vi "Fetch Measurement (Harmonic Distortion).vi"(8 "error in (no error)":errorcluster, 9 "Timeout (20000 ms)":i32=20000, 11 "VISA resource name":refnum<visa-resource-name>) -> (0 "error out":errorcluster, 1 "Frequency Values":dbl[](array[numeric]) format="%#.6g", 2 "Amplitude Values":dbl[](array[numeric]) format="%#.6g", 3 "VISA resource name out":refnum<visa-resource-name>, 5 "Frequency Of The Fundamental (Hz)":dbl format="%#.6g", 7 "Total Harmonic Distortion":dbl format="%#.6g")   [LabVIEW 2014, in "Agilent ESA PSA Series.lvlib"]
doc: "Returns the results of the last measurement(Harmonic Distortion) and does not initiate data acquisition."
uses:
  Agilent ESA PSA Series.lvlib
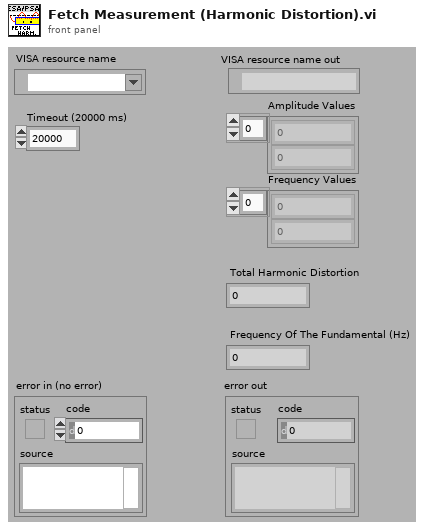
[diagram p1: front panel]
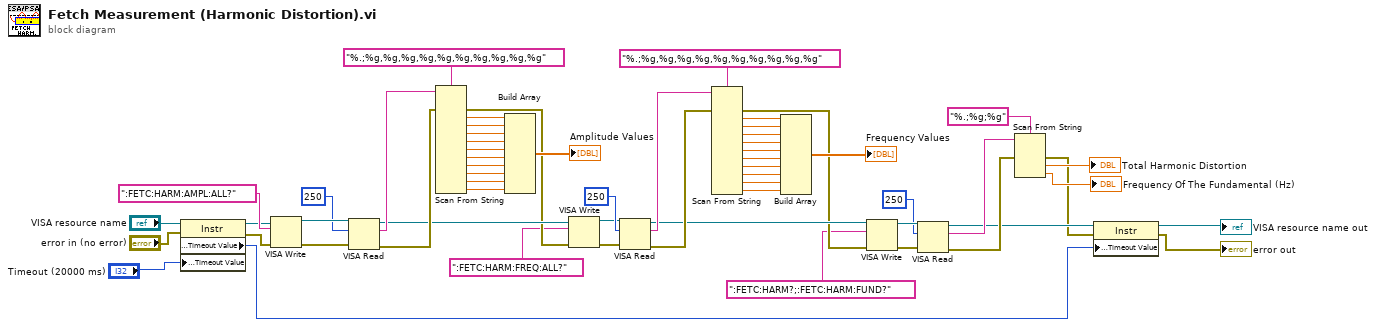
[diagram p0: block diagram]
diagram:
  n1 = property on="Property Node" class="Instr"(reference="VISA resource name", error in="error in (no error)", "General Settings:Timeout Value"="Timeout (20000 ms)") -> (reference out=w8:refnum<visa-resource-name>, error out=w7:errorcluster, "General Settings:Timeout Value"=w4:u32)
  n2 = VISA Write(VISA resource name=w8, write buffer=":FETC:HARM:AMPL:ALL?", error in (no error)=w7) -> (VISA resource name out=w48:refnum<visa-resource-name>, error out=w46:errorcluster)  [unwired: 1 out]
  n3 = VISA Read(VISA resource name=w48, byte count=u32 250, error in (no error)=w46) -> (VISA resource name out=w38:refnum<visa-resource-name>, read buffer=w45:string, error out=w42:errorcluster)  [unwired: 1 out]
  n4 = Scan From String(format string="%.;%g,%g,%g,%g,%g,%g,%g,%g,%g,%g", input string=w45, error in=w42) -> (error out=w37:errorcluster, output 1=w57:dbl, output 2=w55:dbl, output 3=w54:dbl, output 4=w53:dbl, output 5=w52:dbl, output 6=w51:dbl, output 7=w50:dbl, output 8=w49:dbl, output 9=w44:dbl, output 10=w43:dbl)  [unwired: 11 in, 2 out]
  n5 = Build Array(w57, w55, w54, w53, w52, w51, w50, w49, w44, w43) -> (→"Amplitude Values":dbl[])
  n6 = VISA Write(VISA resource name=w38, write buffer=":FETC:HARM:FREQ:ALL?", error in (no error)=w37) -> (VISA resource name out=w39:refnum<visa-resource-name>, error out=w41:errorcluster)  [unwired: 1 out]
  n7 = VISA Read(VISA resource name=w39, byte count=u32 250, error in (no error)=w41) -> (VISA resource name out=w18:refnum<visa-resource-name>, read buffer=w23:string, error out=w22:errorcluster)  [unwired: 1 out]
  n8 = Scan From String(format string="%.;%g,%g,%g,%g,%g,%g,%g,%g,%g,%g", input string=w23, error in=w22) -> (error out=w17:errorcluster, output 1=w25:dbl, output 2=w27:dbl, output 3=w28:dbl, output 4=w29:dbl, output 5=w30:dbl, output 6=w31:dbl, output 7=w32:dbl, output 8=w33:dbl, output 9=w34:dbl, output 10=w35:dbl)  [unwired: 11 in, 2 out]
  n9 = Build Array(w25, w27, w28, w29, w30, w31, w32, w33, w34, w35) -> (→"Frequency Values":dbl[])
  n10 = VISA Write(VISA resource name=w18, write buffer=":FETC:HARM?;:FETC:HARM:FUND?", error in (no error)=w17) -> (VISA resource name out=w21:refnum<visa-resource-name>, error out=w19:errorcluster)  [unwired: 1 out]
  n11 = VISA Read(VISA resource name=w21, byte count=u32 250, error in (no error)=w19) -> (VISA resource name out=w6:refnum<visa-resource-name>, read buffer=w14:string, error out=w13:errorcluster)  [unwired: 1 out]
  n12 = Scan From String(format string="%.;%g;%g", input string=w14, error in=w13) -> (error out=w5:errorcluster, output 1=→"Total Harmonic Distortion":dbl, output 2=→"Frequency Of The Fundamental (Hz)":dbl)  [unwired: 3 in, 2 out]
  n13 = property on="Property Node" class="Instr"(reference=w6, error in=w5, "General Settings:Timeout Value"=w4) -> (reference out=→"VISA resource name out":refnum<visa-resource-name>, error out=→"error out":errorcluster)
